vi "sub_ofdm_subcarrier_allocator.vi"(8 "fft size":i32=256, 9 "pilot symbol":cdb[](array[numeric]), 11 "message symbol":cdb[](array[numeric])) -> (3 "OFDM symbol":cdb[](array[numeric]))   [LabVIEW 2014]
panel:
  out "positive freq size":i32
  out "negative freq size":i32
  out "DC term previous":cdb
  out "DC term next":cdb
  out "DC term":cdb
  out "size(s)":i32
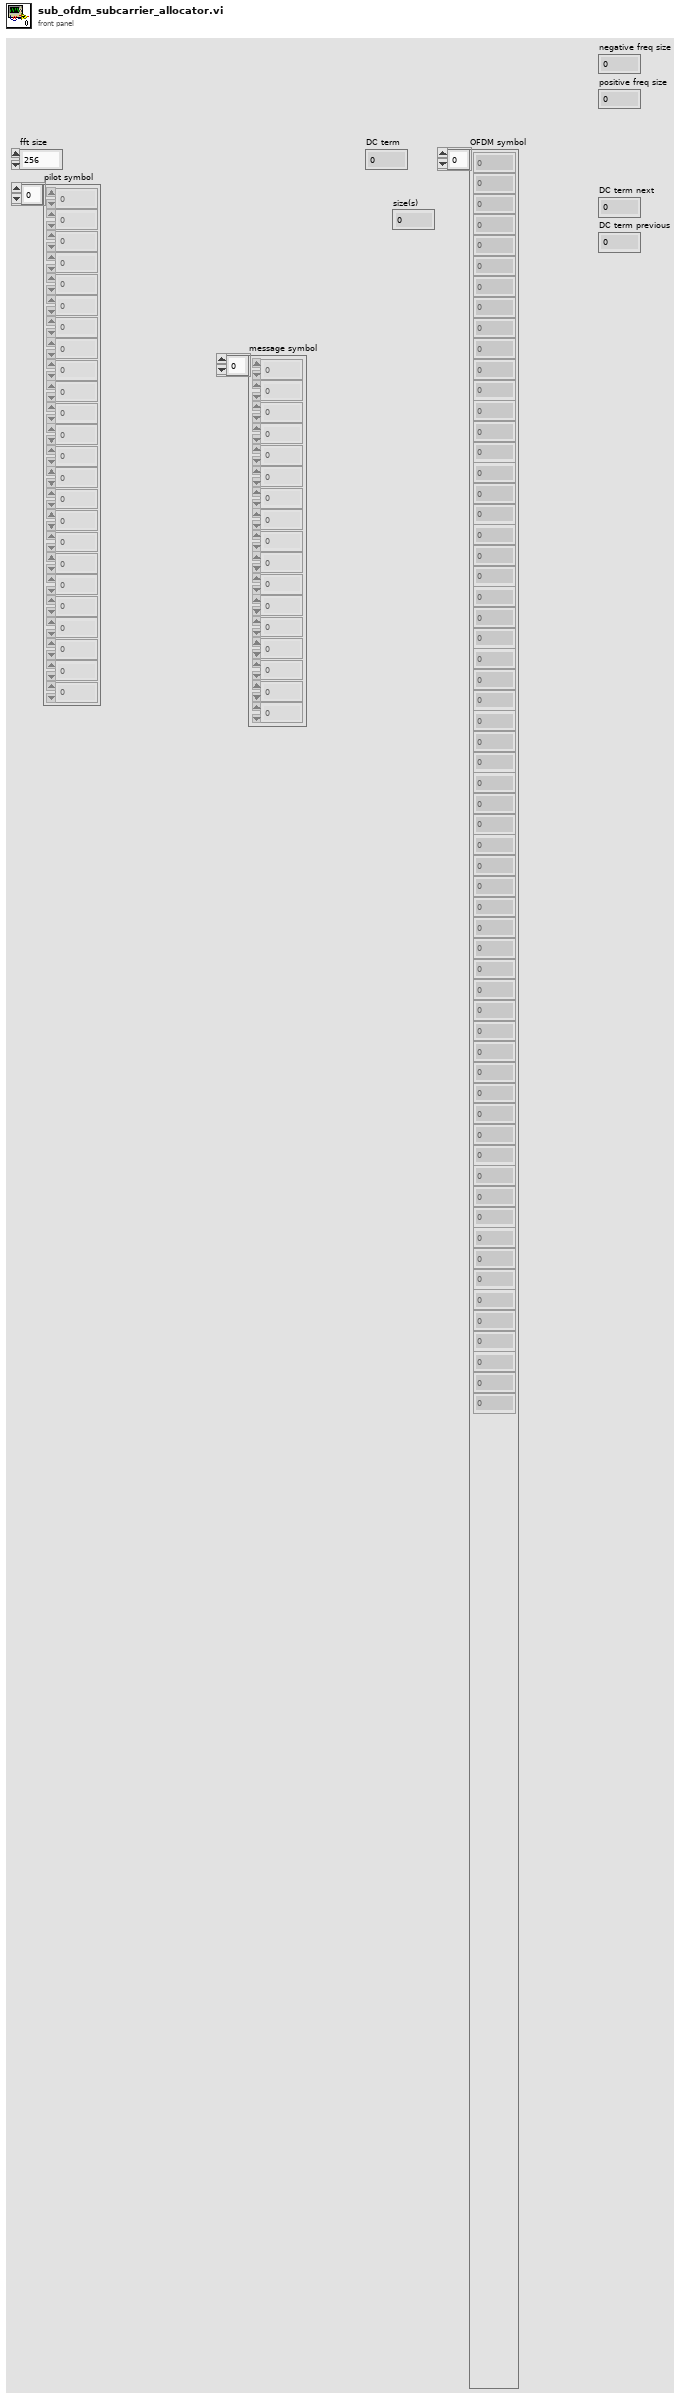
[diagram p1: front panel]
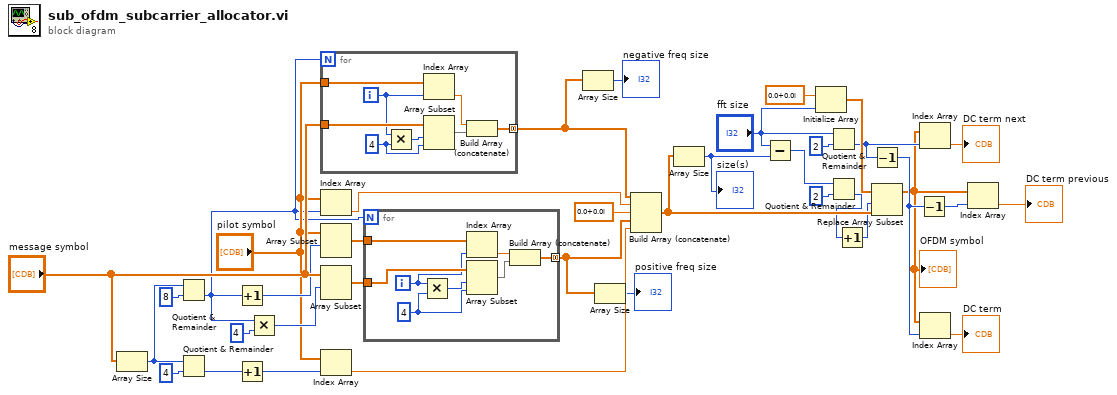
[diagram p0: block diagram]
diagram:
  n1 = Array Size(array="message symbol") -> (size(s)=w25:i32)
  n2 = Quotient & Remainder(x=w25, y=8) -> (floor(x/y)=w19:i32)  [unwired: 1 out]
  n3 = Quotient & Remainder(x=w25, y=4) -> (floor(x/y)=w20:i32)  [unwired: 1 out]
  n4 = Increment(x=w19) -> (x+1=w29:i32)
  n5 = Increment(x=w20) -> (x+1=w23:i32)
  n6 = Multiply(x=w19, y=4) -> (x*y=w31:i32)
  n7 = for {
    N: w19 -> [_]
    tunnel: "message symbol" -> [w43]
    tunnel: "pilot symbol" -> [w42]
    tunnel: [w38] -> w6 mode=concatenating
    i -> [w41]
    w45 = 4
    n8 = Multiply(x=w41, y=w45) -> (x*y=w44:i32)
    n9 = Index Array(array=w42, index=w41) -> (element=w40:cdb)
    n10 = Array Subset(array=w43, index=w44, length=w45) -> (w39:cdb[])
    n11 = Build Array (concatenate)(w40, w39) -> (w38:cdb[])
  }
  n12 = Index Array(array="pilot symbol", index=w19) -> (element=w35:cdb)
  n13 = Array Subset(array="pilot symbol", index=w29) -> (w28:cdb[])  [unwired: 1 in]
  n14 = Array Subset(array="message symbol", index=w31) -> (w30:cdb[])  [unwired: 1 in]
  n15 = Index Array(array="pilot symbol", index=w23) -> (element=w27:cdb)
  n16 = for {
    N: w19 -> [_]
    tunnel: w30 -> [w51]
    tunnel: w28 -> [w50]
    tunnel: [w46] -> w4 mode=concatenating
    i -> [w49]
    w53 = 4
    n17 = Multiply(x=w49, y=w53) -> (x*y=w52:i32)
    n18 = Index Array(array=w50, index=w49) -> (element=w48:cdb)
    n19 = Array Subset(array=w51, index=w52, length=w53) -> (w47:cdb[])
    n20 = Build Array (concatenate)(w48, w47) -> (w46:cdb[])
  }
  n21 = Array Size(array=w6) -> (size(s)=→"negative freq size":i32)
  n22 = Array Size(array=w4) -> (size(s)=→"positive freq size":i32)
  n23 = Build Array (concatenate)(w6, w35, cdb 0.0+0.0i, w4, w27) -> (w21:cdb[])
  n24 = Array Size(array=w21) -> (size(s)=w18:i32)
  "size(s)" <- w18
  n25 = Subtract(x="fft size", y=w18) -> (x-y=w17:i32)
  n26 = Initialize Array(cdb 0.0+0.0i, "fft size") -> (w22:cdb[])
  n27 = Quotient & Remainder(x="fft size", y=2) -> (floor(x/y)=w12:i32)  [unwired: 1 out]
  n28 = Quotient & Remainder(x=w17, y=2) -> (floor(x/y)=w2:i32)  [unwired: 1 out]
  n29 = Increment(x=w2) -> (x+1=w1:i32)
  n30 = Decrement(x=w12) -> (x-1=w10:i32)
  n31 = Replace Array Subset(array=w22, new element=w21, index=w1) -> (w8:cdb[])
  "OFDM symbol" <- w8
  n32 = Decrement(x=w10) -> (x-1=w9:i32)
  n33 = Index Array(array=w8, index=w12) -> (element=→"DC term next":cdb)
  n34 = Index Array(array=w8, index=w10) -> (element=→"DC term":cdb)
  n35 = Index Array(array=w8, index=w9) -> (element=→"DC term previous":cdb)
